vi "17-FindVx.vi"(11 "Target in":T2) -> (2 "x Velocity Info":T1(array[cluster]), 3 "Target out":T2)   [LabVIEW 2019, in "17.lvlib"]
uses:
  17.lvlib
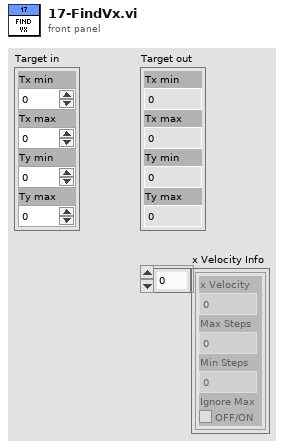
[diagram p1: front panel]
types:
  T1 = cluster{"x Velocity":i32, "Max Steps":i32, "Min Steps":i32, "Ignore Max":bool}[]
  T2 = cluster{"Tx min":i32, "Tx max":i32, "Ty min":i32, "Ty max":i32}
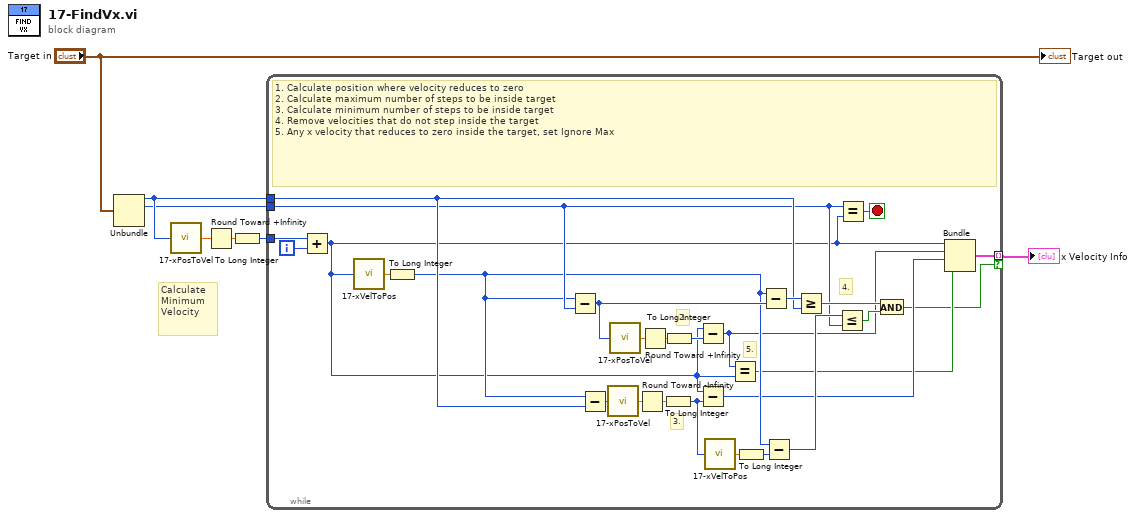
[diagram p0: block diagram]
diagram:
  # "Calculate Minimum \nVelocity"
  n1 = Unbundle("Target in") -> ("Tx min"=w6:i32, "Tx max"=w5:i32)  [unwired: 2 out]
  n2 = call "17-xPosToVel.vi"("x position"=w6) -> ("x velocity"=w3:dbl)
  n3 = Round Toward +Infinity(x=w3) -> (ceil(x): smallest int >= x=w4:dbl)
  n4 = To Long Integer(number=w4) -> (32bit integer=w7:i32)
  n5 = while {
    tunnel: w5 -> [w22]
    tunnel: w6 -> [w31]
    tunnel: [w12] -> w1 mode=indexing if=w11
    tunnel: w7 -> [w10]
    i -> [w8]
    stop <- w21 stop-if-true
    # "5."
    # "4."
    # "3."
    # "2."
    # "1. Calculate position where velocity reduces to zero\n2. Calculate maximum number of steps to be inside target\n3. Calculate minimum number of steps to be inside target \n4. Remove velocities that do not step inside the target\n5. Any x velocity that reduces to zero inside the target, set Ignore Max"
    n6 = Add(x=w10, y=w8) -> (x+y=w9:i32)
    n7 = call "17-xVelToPos.vi"("x velocity"=w9) -> ("x position"=w26:dbl)
    n8 = To Long Integer(number=w26) -> (32bit integer=w19:i32)
    n9 = Subtract(x=w19, y=w22) -> (x-y=w20:i32)
    n10 = Subtract(x=w19, y=w31) -> (x-y=w28:i32)
    n11 = call "17-xPosToVel.vi"("x position"=w28) -> ("x velocity"=w27:dbl)
    n12 = call "17-xPosToVel.vi"("x position"=w20) -> ("x velocity"=w34:dbl)
    n13 = Round Toward -Infinity(1:w27) -> (0:w25:dbl)
    n14 = Round Toward +Infinity(x=w34) -> (ceil(x): smallest int >= x=w33:dbl)
    n15 = To Long Integer(number=w25) -> (32bit integer=w17:i32)
    n16 = To Long Integer(number=w33) -> (32bit integer=w16:i32)
    n17 = Subtract(x=w9, y=w16) -> (x-y=w15:i32)
    n18 = Subtract(x=w9, y=w17) -> (x-y=w14:i32)
    n19 = call "17-xVelToPos.vi"("x velocity"=w17) -> ("x position"=w24:dbl)
    n20 = Equal?(x=w15, y=w9) -> (x = y?=w13:bool)
    n21 = To Long Integer(number=w24) -> (32bit integer=w18:i32)
    n22 = Subtract(x=w19, y=w20) -> (x-y=w32:i32)
    n23 = Subtract(x=w19, y=w18) -> (x-y=w30:i32)
    n24 = Greater Or Equal?(x=w32, y=w31) -> (x >= y?=w23:bool)
    n25 = Less Or Equal?(x=w30, y=w22) -> (x <= y?=w29:bool)
    n26 = Equal?(x=w22, y=w9) -> (x = y?=w21:bool)
    n27 = And(x=w23, y=w29) -> (x .and. y?=w11:bool)
    n28 = Bundle(w9, w15, w14, w13) -> (w12:cluster{i32, i32, i32, bool})  [unwired: 1 in]
  }
  "x Velocity Info" <- w1
  "Target out" <- "Target in"
